vi "Rectangle match to ROI.vi"(8 "error in (no error)":errorcluster, 11 "Rectangles":T1(array[cluster])) -> (0 "error out":errorcluster, 3 "ROI Descriptor":T2 {"Contours"."Type" items=["No Selection", "Point", "Line", "Rectangle", "Oval", "Polygon", "Freehand Region", "Annulus", "Unused2", "Unused3", "Broken Line", "Freehand Line", "Rotated Rectangle"]})   [LabVIEW 2018]
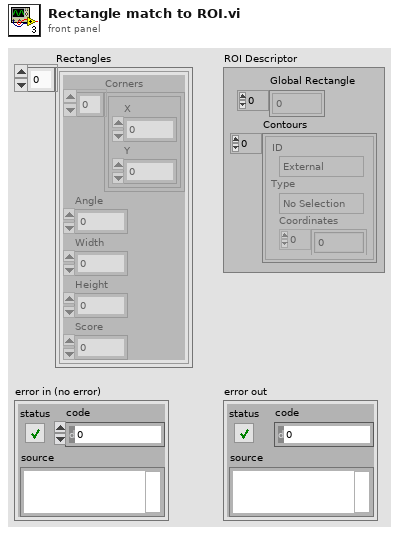
[diagram p1: front panel]
types:
  T1 = cluster{"Corners":cluster{"X":sgl, "Y":sgl}[], "Angle":dbl, "Width":dbl, "Height":dbl, "Score":dbl}[]
  T2 = typedef "ROI Descriptor" = cluster{"Global Rectangle":i32[], "Contours":cluster{"ID":enum32{"External", "Internal"}, "Type":u32, "Coordinates":i32[]}[]}
  T3 = typedef "IMAQ Rectangle" = cluster{"Left":i32, "Top":i32, "Right":i32, "Bottom":i32, "Rotation":dbl}
  T4 = cluster{"Corners":cluster{"X":sgl, "Y":sgl}[], "Angle":dbl, "Width":dbl, "Height":dbl, "Score":dbl}
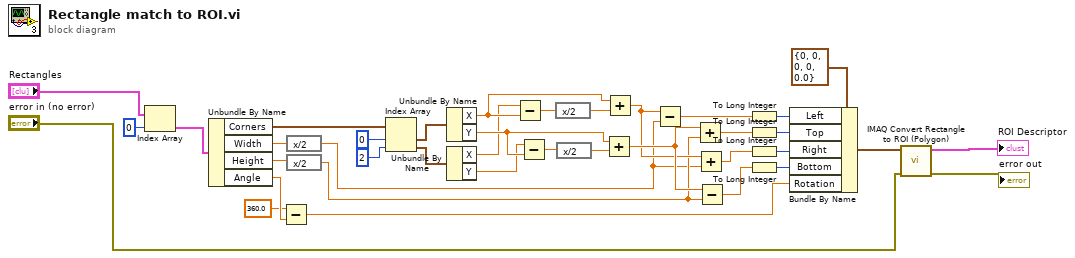
[diagram p0: block diagram]
diagram:
  n1 = Index Array(array="Rectangles", index=0) -> (element=w1:T4)
  n2 = Unbundle By Name(w1) -> ("Corners"=w4:cluster{"X":sgl, "Y":sgl}[], "Width"=w16:dbl, "Height"=w17:dbl, "Angle"=w15:dbl)
  n3 = Subtract(x=360.0, y=w15) -> (x-y=w10:dbl)
  n4 = expression code="x/2"(w16) -> (w18:dbl)
  n5 = expression code="x/2"(w17) -> (w19:dbl)
  n6 = Index Array(array=w4, index #1=0 ("index"), index #2=2 ("index")) -> (element #1=w5:cluster{"X":sgl, "Y":sgl}, element #2=w8:cluster{"X":sgl, "Y":sgl})
  n7 = Unbundle By Name(w5) -> ("X"=w21:sgl, "Y"=w24:sgl)
  n8 = Unbundle By Name(w8) -> ("X"=w11:sgl, "Y"=w12:sgl)
  n9 = Subtract(x=w11, y=w21) -> (x-y=w13:sgl)
  n10 = Subtract(x=w12, y=w24) -> (x-y=w14:sgl)
  n11 = expression code="x/2"(w13) -> (w22:sgl)
  n12 = expression code="x/2"(w14) -> (w25:sgl)
  n13 = Add(x=w24, y=w25) -> (x+y=w23:sgl)
  n14 = Add(x=w21, y=w22) -> (x+y=w20:sgl)
  n15 = Subtract(x=w20, y=w18) -> (x-y=w30:dbl)
  n16 = Add(x=w23, y=w19) -> (x+y=w31:dbl)
  n17 = Add(x=w20, y=w18) -> (x+y=w32:dbl)
  n18 = Subtract(x=w23, y=w19) -> (x-y=w33:dbl)
  n19 = To Long Integer(number=w30) -> (32bit integer=w26:i32)
  n20 = To Long Integer(number=w31) -> (32bit integer=w27:i32)
  n21 = To Long Integer(number=w32) -> (32bit integer=w28:i32)
  n22 = To Long Integer(number=w33) -> (32bit integer=w29:i32)
  n23 = Bundle By Name(cluster=T3 {"Left"=0, "Top"=0, "Right"=0, "Bottom"=0, "Rotation"=0.0} ("Rectangle"), "Left"=w26, "Top"=w27, "Right"=w28, "Bottom"=w29, "Rotation"=w10) -> (w35:T3)
  n24 = call "IMAQ Convert Rectangle to ROI (Polygon)"("error in (no error)"="error in (no error)", "Rectangle"=w35) -> ("error out"=→"error out":errorcluster, "ROI Descriptor"=→"ROI Descriptor":T2)  [unwired: 6 in, 1 out]
